vi "crearTupla.vi"(5 "clusterMetalRodDataIn":T1, 6 "clusterProductDataIn":T3, 7 "clusterStadisticDataIn":T2, 8 "tableName":string, 9 "clusterRecipeDataIn":T4, 10 "clusterImageDataIn":T5, 11 "error in":errorcluster) -> (3 "error out":errorcluster)   [LabVIEW 2014]
uses:
  <vilib>/addons/database/Connection.llb/DB Tools Open Connec (String).vi
  <vilib>/addons/database/NI_Database_API.lvlib
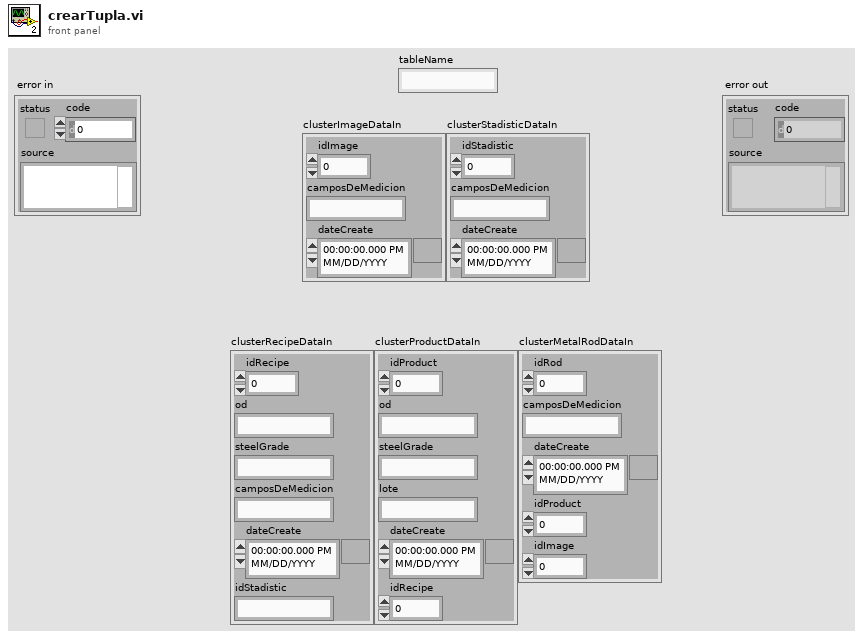
[diagram p1: front panel]
types:
  T1 = cluster{"idRod":dbl, "camposDeMedicion":string, "dateCreate":timestamp, "idProduct":dbl, "idImage":dbl}
  T2 = cluster{"idStadistic":dbl, "camposDeMedicion":string, "dateCreate":timestamp}
  T3 = cluster{"idProduct":dbl, "od":string, "steelGrade":string, "lote":string, "dateCreate":timestamp, "idRecipe":dbl}
  T4 = cluster{"idRecipe":dbl, "od":string, "steelGrade":string, "camposDeMedicion":string, "dateCreate":timestamp, "idStadistic":string}
  T5 = cluster{"idImage":dbl, "camposDeMedicion":string, "dateCreate":timestamp}
  T6 = typedef "NI_Database_API.lvlib/Conn ObjectReference.ctl" = refnum<k1>
  T7 = typedef "NI_Database_API.lvlib/DB Tools DataTypes.ctl" = enum16{"String", "Long (I32)", "Single (SGL)", "Double (DBL)", "Date/Time", "Binary"}
  T8 = cluster{"name":string, "database data type":T7, "defined size":i32}[]
  T9 = cluster{string, "od":string, "steelGrade":string, "camposDeMedicion":string, "date/time string":string}
  T10 = cluster{string, "od":string, "steelGrade":string, "lote":string, "date/time string":string}
  T11 = cluster{string, "camposDeMedicion":string, "date/time string":string}
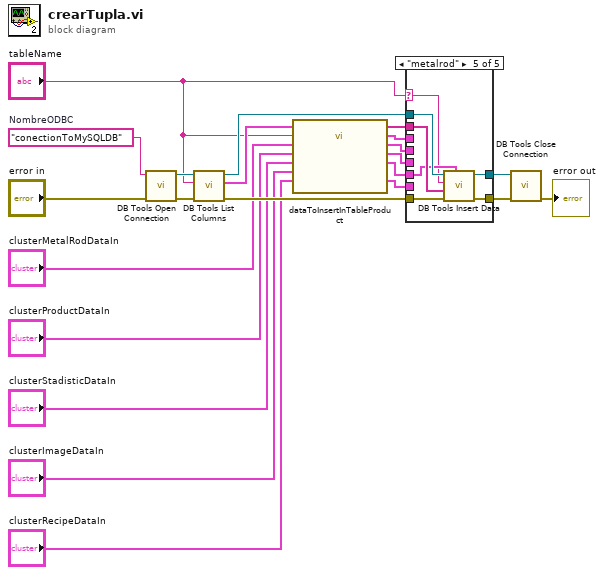
[diagram p0: block diagram]
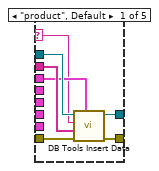
[diagram p2: hidden frame]
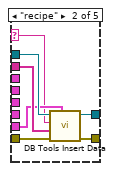
[diagram p3: hidden frame]
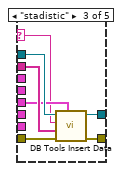
[diagram p4: hidden frame]
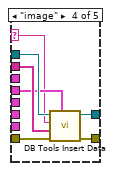
[diagram p5: hidden frame]
diagram:
  w22 = "conectionToMySQLDB"  # NombreODBC
  n1 = call-poly <vilib>:"DB Tools Open Connection.vi"("error in (no error)"="error in", "connection information"=w22) -> ("error out"=w12:errorcluster, "connection reference"=w13:T6)  [unwired: 6 in]
  n2 = call <vilib>:"DB Tools List Columns.vi"("error in (no error)"=w12, "table"="tableName", "connection reference"=w13) -> ("error out"=w20:errorcluster, "column information"=w19:T8, "connection reference out"=w21:T6)  [unwired: 1 in, 1 out]
  n3 = call "dataToInsertInTableProduct.vi"("arrayNamesInTableIN"=w19, "clusterRecipeDataIn"="clusterRecipeDataIn", "clusterImageDataIn"="clusterImageDataIn", "tableIn"="tableName", "clusterMetalRodDataIn"="clusterMetalRodDataIn", "clusterProductDataIn"="clusterProductDataIn", "clusterStadisticDataIn"="clusterStadisticDataIn") -> ("clusterRecipeDataOut"=w17:T9, "arrayNamesInTableOUT"=w14:string[], "clusterProductDataOut"=w16:T10, "clusterImageDataOut"=w18:T11, "clusterMetalRodDataOut"=w15:T11, "clusterStadisticDataOut"=w9:T11)  [unwired: 2 in, 1 out]
  n4 = case shown="\"metalrod\"" "tableName" {
    selector: "tableName" -> [w23 w30 w37 w44 w51]
    tunnel: w21 -> [w29 w36 w43 w50 w57]
    tunnel: w20 -> [w27 w35 w41 w48 w56]
    tunnel: [w26 w34 w42 w49 w55] -> w11
    tunnel: [w25 w33 w40 w47 w54] -> w10
    tunnel: w14 -> [w28 w32 w39 w46 w53]
    tunnel: w15 -> [_ _ _ _ w52]
    tunnel: w16 -> [w24 _ _ _ _]
    tunnel: w17 -> [_ w31 _ _ _]
    tunnel: w9 -> [_ _ w38 _ _]
    tunnel: w18 -> [_ _ _ w45 _]
    frame "product", Default {
      n5 = call <vilib>:"DB Tools Insert Data.vi"("data"=w24, "error in (no error)"=w27, "columns"=w28, "table"=w23, "connection reference"=w29) -> ("error out"=w25:errorcluster, "connection reference out"=w26:T6)  [unwired: 5 in]
    }
    frame "recipe" {
      n6 = call <vilib>:"DB Tools Insert Data.vi"("data"=w31, "error in (no error)"=w35, "columns"=w32, "table"=w30, "connection reference"=w36) -> ("error out"=w33:errorcluster, "connection reference out"=w34:T6)  [unwired: 5 in]
    }
    frame "stadistic" {
      n7 = call <vilib>:"DB Tools Insert Data.vi"("data"=w38, "error in (no error)"=w41, "columns"=w39, "table"=w37, "connection reference"=w43) -> ("error out"=w40:errorcluster, "connection reference out"=w42:T6)  [unwired: 5 in]
    }
    frame "image" {
      n8 = call <vilib>:"DB Tools Insert Data.vi"("data"=w45, "error in (no error)"=w48, "columns"=w46, "table"=w44, "connection reference"=w50) -> ("error out"=w47:errorcluster, "connection reference out"=w49:T6)  [unwired: 5 in]
    }
    frame "metalrod" {
      n9 = call <vilib>:"DB Tools Insert Data.vi"("data"=w52, "error in (no error)"=w56, "columns"=w53, "table"=w51, "connection reference"=w57) -> ("error out"=w54:errorcluster, "connection reference out"=w55:T6)  [unwired: 5 in]
    }
  }
  n10 = call <vilib>:"DB Tools Close Connection.vi"("error in (no error)"=w10, "connection reference"=w11) -> ("error out"=→"error out":errorcluster)  [unwired: 5 in]
